vi "check cluster field names.vi"(8 "error in (no error)":errorcluster, 11 "cluster or arr in":variant) -> (0 "error out":errorcluster)   [LabVIEW 2018, in "LV-0mq-Julia_roundtrip-lib.lvlib" / "LV2Julia_core.lvlib"]
uses:
  LV2Julia_core.lvlib
  <vilib>/Utility/error.llb/Error Cluster From Error Code.vi
  <vilib>/ErrorRing/Error Ring.xnode
  <vilib>/Utility/Data Type/NI_Data Type.lvlib
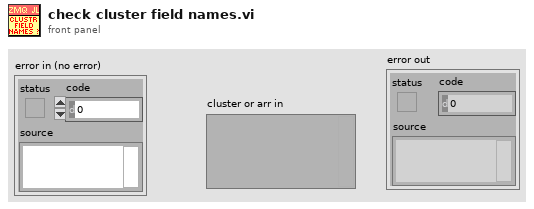
[diagram p1: front panel]
types:
  T1 = typedef "NI_Data Type.lvlib/Data Type.ctl" = enum8{"Invalid Type", "Void", "I8", "I16", "I32", "I64", "U8", "U16", "U32", "U64", "Single Float", "Double Float", "Extended Float", "Single Complex", "Double Complex", "Extended Complex", "Enum U8", "Enum U16", "Enum U32", "Enum U64", "Single Float With Unit", "Double Float With Unit", "Extended Float With Unit", "Single Complex with Unit", "Double Complex with Unit", "Extended Complex with Unit", "Boolean", "String", "Path", "Picture", "Tag", "Array", "Cluster", "Variant", "LV Variant", "Waveform", "Timestamp", "Digital Waveform", "Digital Data", "ExpressData", "Refnum", "External Data", "VI", "Poly VI", "LabVIEW Class Instance", "Fixed Point"}
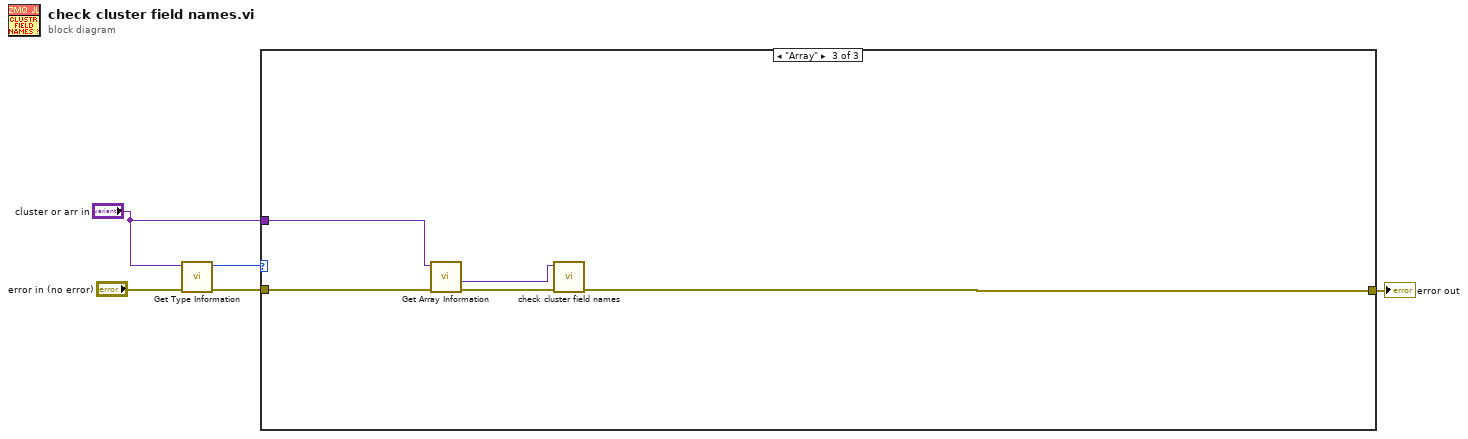
[diagram p0: block diagram]
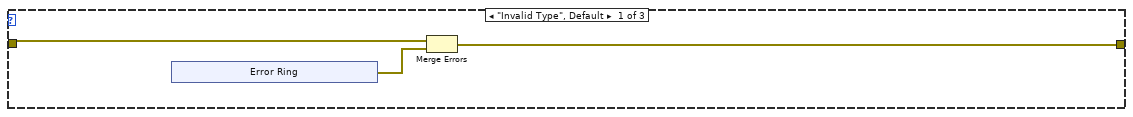
[diagram p2: hidden frame]
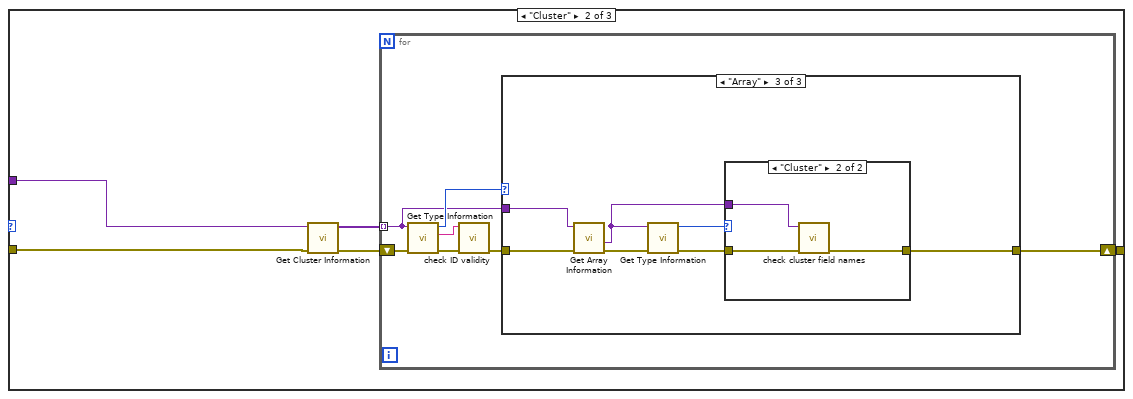
[diagram p3: hidden frame]
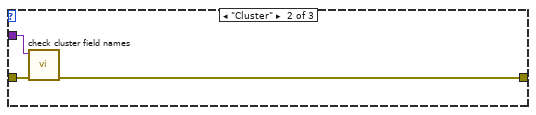
[diagram p5: hidden frame]
diagram:
  n1 = call <vilib>:"Get Type Information.vi"("error in (no error)"="error in (no error)", "Variant"="cluster or arr in") -> ("error out"=w2:errorcluster, "Type"=w3:T1)  [unwired: 5 in, 3 out]
  n2 = case shown="\"Array\"" w3 {
    tunnel: [w6 w16 w42] -> w5
    tunnel: w2 -> [w7 w15 w45]
    tunnel: "cluster or arr in" -> [_ w14 w44]
    frame "Invalid Type", Default {
      n3 = xnode "Error Ring"() -> ("error out"=w8:errorcluster)
      n4 = Merge Errors(w7, w8) -> (w6:errorcluster)
    }
    frame "Cluster" {
      n5 = call <vilib>:"Get Cluster Information.vi"("error in (no error)"=w15, "Variant"=w14) -> ("error out"=w17:errorcluster, "Cluster Elements"=w18:variant[])  [unwired: 8 in]
      n6 = for {
        tunnel: w18 -> [w19] mode=indexing
        shift-right: [w21] -> w16
        shift-left: w17 -> [w25]
        n7 = call <vilib>:"Get Type Information.vi"("error in (no error)"=w25, "Variant"=w19) -> ("error out"=w24:errorcluster, "Name"=w23:string, "Type"=w20:T1)  [unwired: 5 in, 2 out]
        n8 = call "check ID validity.vi"("error in (no error)"=w24, "ID in"=w23) -> ("error out"=w22:errorcluster)  [unwired: 8 in, 1 out]
        n9 = case shown="\"Array\"" w20 {
          tunnel: [w26 w28 w33] -> w21
          tunnel: w22 -> [w26 w29 w36]
          tunnel: w19 -> [_ w27 w35]
          frame "Invalid Type", Default {
          }
          frame "Cluster" {
            n10 = call "check cluster field names.vi"("error in (no error)"=w29, "cluster or arr in"=w27) -> ("error out"=w28:errorcluster)  [unwired: 9 in]
          }
          frame "Array" {
            n11 = call <vilib>:"Get Array Information.vi"("error in (no error)"=w36, "Variant"=w35) -> ("error out"=w34:errorcluster, "Array Element Data Type"=w30:variant)  [unwired: 6 in, 2 out]
            n12 = call <vilib>:"Get Type Information.vi"("error in (no error)"=w34, "Variant"=w30) -> ("error out"=w32:errorcluster, "Type"=w31:T1)  [unwired: 5 in, 3 out]
            n13 = case shown="\"Cluster\"" w31 {
              tunnel: [w37 w40] -> w33
              tunnel: w32 -> [w37 w39]
              tunnel: w30 -> [_ w38]
              frame "I8", Default {
              }
              frame "Cluster" {
                n14 = call "check cluster field names.vi"("error in (no error)"=w39, "cluster or arr in"=w38) -> ("error out"=w40:errorcluster)  [unwired: 9 in]
              }
            }
          }
        }
      }
    }
    frame "Array" {
      n15 = call <vilib>:"Get Array Information.vi"("error in (no error)"=w45, "Variant"=w44) -> ("error out"=w43:errorcluster, "Array Element Data Type"=w41:variant)  [unwired: 6 in, 2 out]
      n16 = call "check cluster field names.vi"("error in (no error)"=w43, "cluster or arr in"=w41) -> ("error out"=w42:errorcluster)  [unwired: 9 in]
    }
  }
  "error out" <- w5
